vi "MS4_demo.vi"() -> ()   [LabVIEW 2012]
uses:
  <vilib>/vision/Image Controls.llb/IMAQ Image.ctl
  <vilib>/Platform/TimedLoop/XDataNode/timing_clust.ctl
  <vilib>/Platform/TimedLoop/XDataNode/nitl_modes.ctl
  <vilib>/Platform/TimedLoop/XDataNode/wakeup.ctl
  <vilib>/FPGAPlugInAG/sbRIO-9636/niLvFpga_Open_sbRIO-9636.vi
  <vilib>/rvi/interface/common/dynamic/niFpgaDynamicAddResources.vi
  Globals.vi
  <vilib>/Utility/error.llb/Error Cluster From Error Code.vi
  <vilib>/rvi/errors/niLvFpgaAdjustHostInterfaceError.vi
  <vilib>/FPGAPlugInAG/Dynamic/niLvFpga_Close_Dynamic.vi
  <vilib>/platform/TimedLoop/XDataNode/XDataNode.xnode
  <vilib>/rvi/interface/nirviOpenFPGA/nirviOpenFPGA.xnode
  FPGA Bitfiles/NIARC_FPGATarget_FPGACompile_yq6Hl1z977U.lvbitx
  <vilib>/rvi/interface/nirviReadWriteControl/nirviReadWriteControl.xnode
  <vilib>/rvi/interface/nirviCloseFPGA/nirviCloseFPGA.xnode
  <vilib>/Platform/TimedLoop/XDataNode/XDNodeRunTimeDep.lvlib
  NiFpgaLv.dll
  <vilib>/rvi/interface/Simulation/niFpgaSimulationCallBeginRW.vi
panel:
  in  "Go to block?":bool
  out "Arm State":enum16{"arm down", "push", "turn", "arm up"}(ring)
  out "Current \nState":T1(ring)
  in  "Claw deadband":dbl
  in  "Block Claw distance":dbl=0.2
  in  "stop":bool
  in  "Enable":bool
  in  "Block Mid Range":dbl=50.0
  in  "Block Y-Offset":dbl=100.0
  in  "Avoid Distance (m)":dbl=0.3
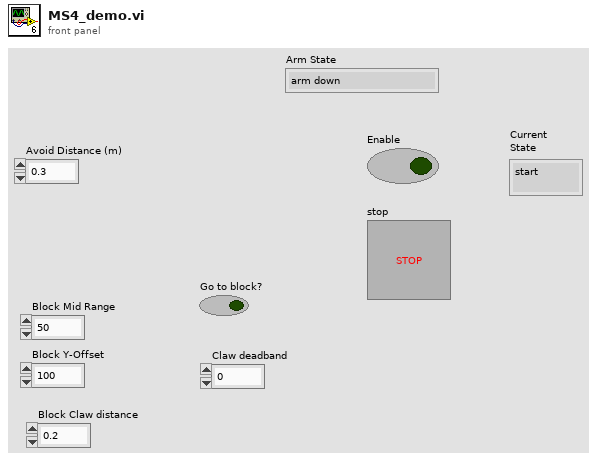
[diagram p1: front panel]
types:
  T1 = enum16{"start", "drive", "turning", "find block", "align block", "pickup"}
  T2 = cluster{"X Velocity (m/s)":dbl, "Y Velocity (m/s)":dbl, "Angular Velocity (rad/s)":dbl}
  T3 = typedef "IMAQ Image.ctl" = refnum<image>
  T4 = typedef "Image Type" = u32
  T5 = enum16{"start", "drive", "turning", "find block", "pickup", ""}
  T6 = enum16{"wait", "open", "close", "lift", "lower", "pickup"}
  T7 = typedef "XDNodeRunTimeDep.lvlib/timing_clust.ctl" = cluster{"Expected End [f-1]":u64, "Actual End [f-1]":u64, "Finished Late? [f-1]":bool, "Expected End [i-1]":u64, "Actual End [i-1]":u64, "Finished Late? [i-1]":bool, "Expected Start [i]":u64, "Actual Start [i]":u64, "Expected Start [f]":u64, "Actual Start [f]":u64, "Source Name":string, "Structure Name":string, "Period":i64, "Deadline":i64, "Offset":i64, "Start":i64, "Priority":i32, "Timeout":i32, "Mode":T8, "Wakeup Reason":T9, "Error":errorcluster, "Source Type":string, "Secondary Source Type":string, "Global End Time":u64, "Global Start Time":u64, "Frame Duration":u64, "Iteration Duration":u64, "Assigned CPU":i32, "I/O Scan Engine Mode":u32}
  T8 = typedef "XDNodeRunTimeDep.lvlib/nitl_modes.ctl" = enum32{"No Change", "Process missed periods, maintain original phase", "Discard missed periods, maintain original phase", "Process missed periods, ignore original phase", "Discard missed periods, ignore original phase"}
  T9 = typedef "XDNodeRunTimeDep.lvlib/wakeup.ctl" = enum32{"Normal", "Aborted", "Asynchronous wakeup", "Timing source error", "Timed loop error", "Timeout"}
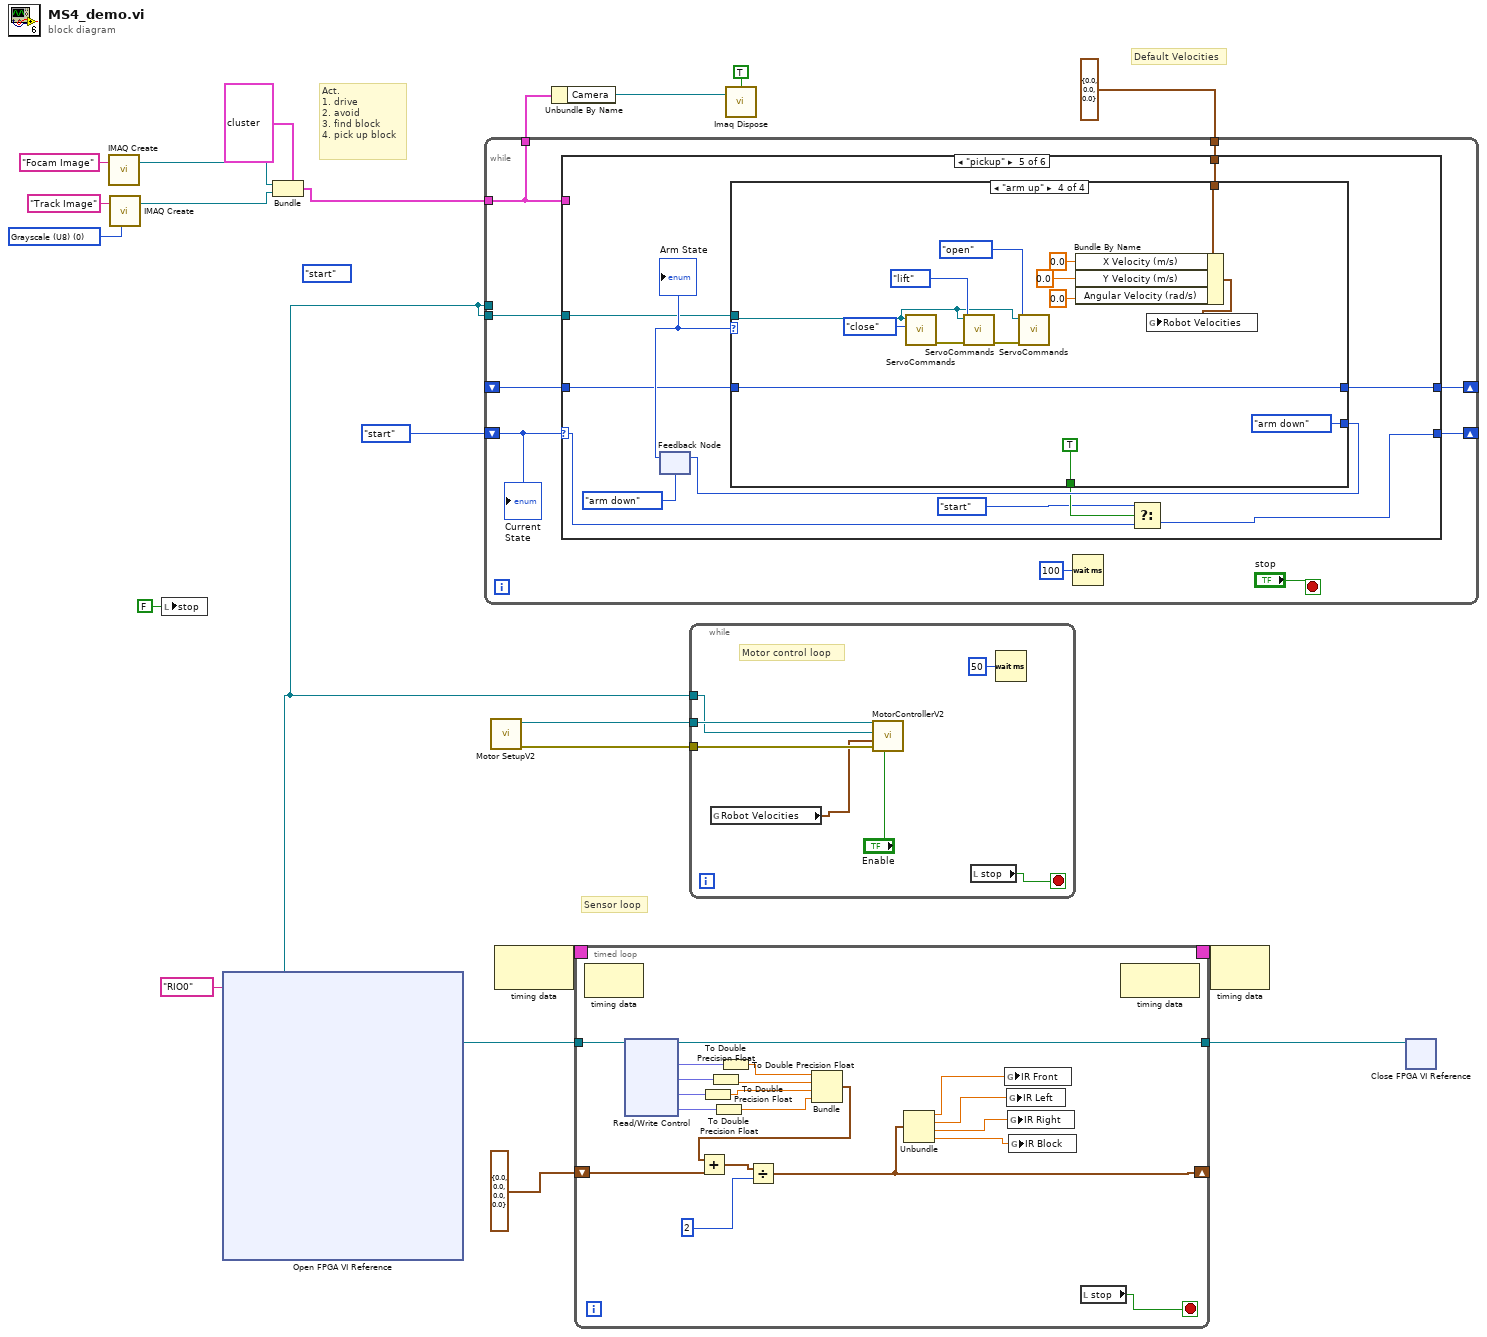
[diagram p0: block diagram]
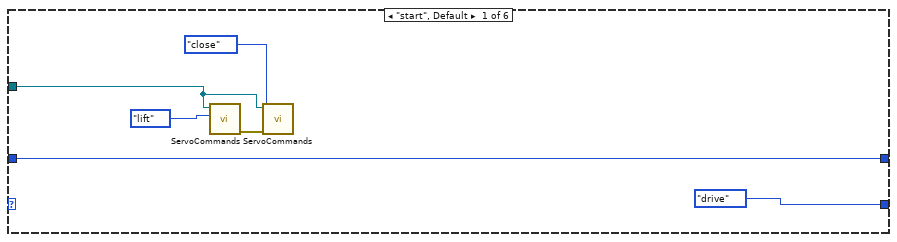
[diagram p2: hidden frame]
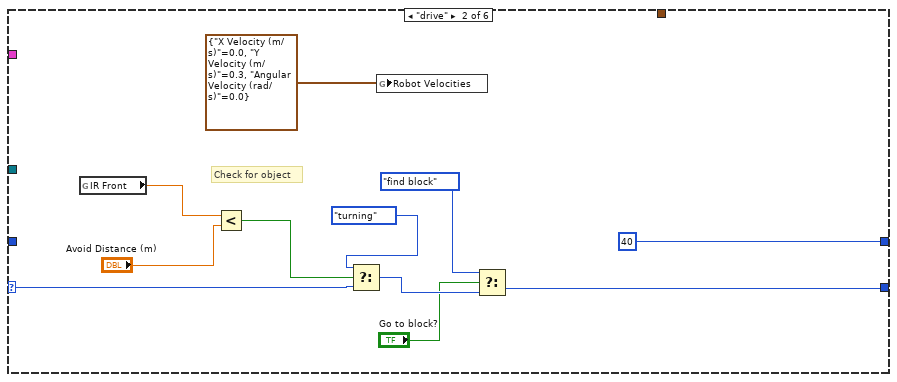
[diagram p3: hidden frame]
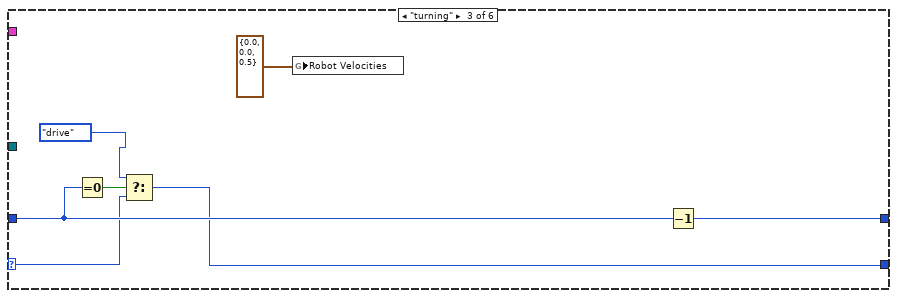
[diagram p4: hidden frame]
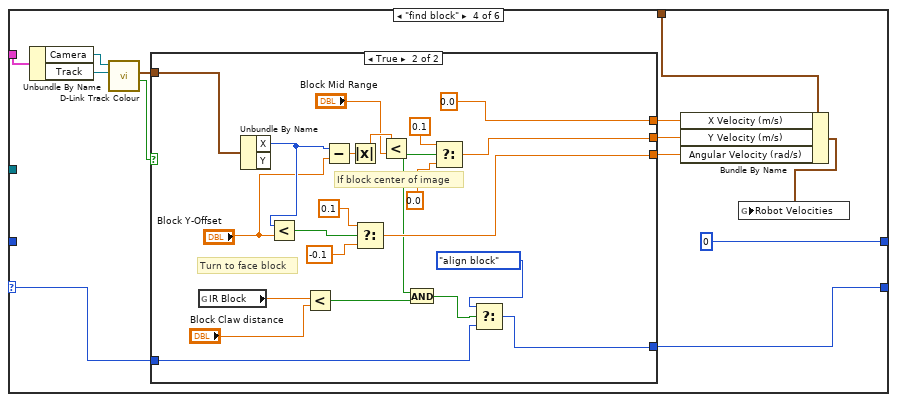
[diagram p5: hidden frame]
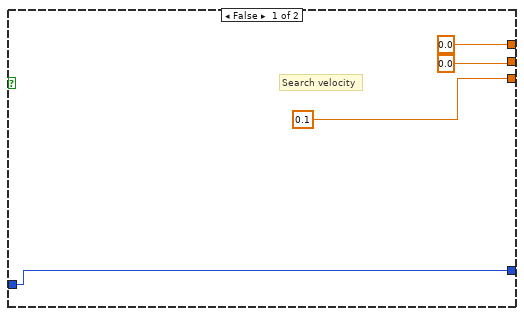
[diagram p6: hidden frame]
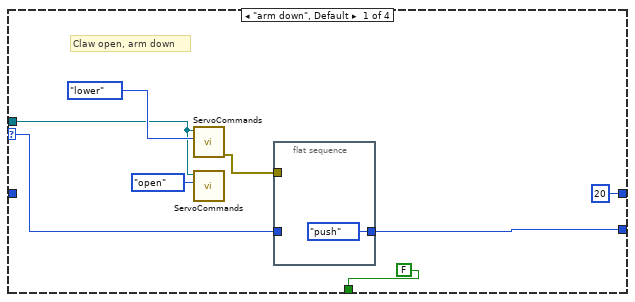
[diagram p7: hidden frame]
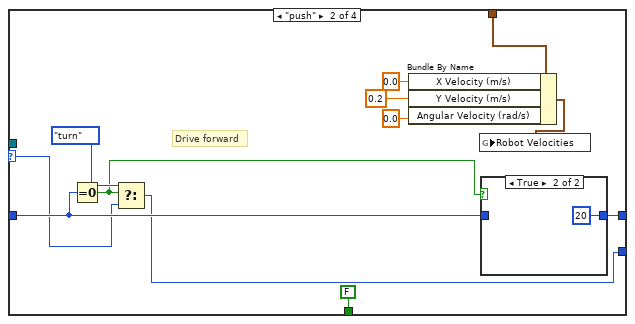
[diagram p8: hidden frame]
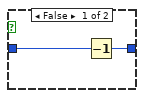
[diagram p9: hidden frame]
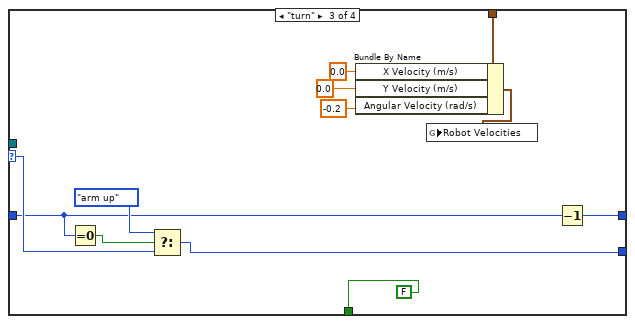
[diagram p10: hidden frame]
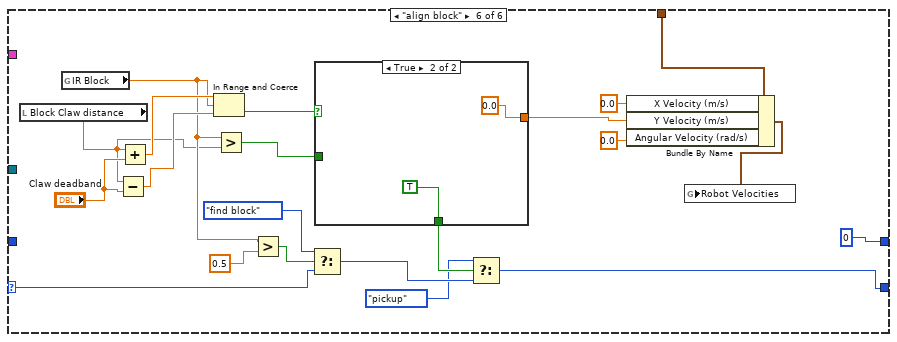
[diagram p11: hidden frame]
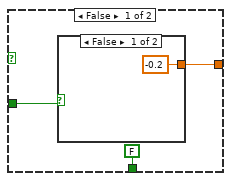
[diagram p12: hidden frame]
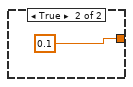
[diagram p13: hidden frame]
diagram:
  w14 = T4 0 items=["Grayscale (U8)", "Grayscale (I16)", "Grayscale (SGL)", "Complex (CSG)", "RGB (U32)", "HSL (U32)", "RGB (U64)", "Grayscale (U16)"] ("Image Type")
  (unwired) T5."start"
  # "Default Velocities"
  # "Sensor loop"
  # "Act.\n1. drive\n2. avoid\n3. find block\n4. pick up block"
  n1 = call "IMAQ Create"("Image Name"="Focam Image") -> ("New Image"=w11:T3)  [unwired: 4 in, 1 out]
  n2 = call "IMAQ Create"("Image Name"="Track Image", "Image Type"=w14) -> ("New Image"=w12:T3)  [unwired: 3 in, 1 out]
  n3 = local write "stop"(FALSE ("stop")) -> ()
  n4 = xnode "Open FPGA VI Reference"("resource name"=tag "RIO0") -> ("FPGA VI Reference Out"=w1:refnum<k20>)  [unwired: 1 in, 1 out]
  n5 = Bundle(cluster=cluster{"Camera":T3, "Track":T3} {"Camera"=refnum, "Track"=refnum}, "Camera"=w11, "Track"=w12) -> (w10:cluster{"Camera":T3, "Track":T3})
  n6 = while {
    tunnel: w1 -> [_]
    shift-right: [w24] -> _
    shift-left: T1."start" -> [w23]
    shift-right: [w30] -> _
    shift-left: _ -> [w29]
    tunnel: w10 -> [w27]
    tunnel: [w27] -> w8
    tunnel: T2 {"X Velocity (m/s)"=0.0, "Y Velocity (m/s)"=0.0, "Angular Velocity (rad/s)"=0.0} ("Robot Velocities") -> [w25]
    tunnel: w1 -> [w22]
    stop <- "stop" stop-if-true
    n7 = case shown="\"pickup\"" w23 {
      selector: w23 -> [_ w44 w51 w56 w97 w161]
      tunnel: [T1."drive" w39 w50 w55 w96 w157] -> w24
      tunnel: [w36 40 w54 0 w100 0] -> w30
      tunnel: w29 -> [w36 _ w53 _ w101 _]
      tunnel: w27 -> [_ _ _ w66 _ _]
      tunnel: w25 -> [_ _ _ w58 w99 w173]
      tunnel: w22 -> [w32 _ _ _ w98 _]
      frame "start", Default {
        n8 = call "ServoCommands.vi"("State"=T6."lift", "FPGA VI Reference In"=w32) -> ("error out"=w33:errorcluster)  [unwired: 9 in]
        n9 = call "ServoCommands.vi"("error in"=w33, "State"=T6."close", "FPGA VI Reference In"=w32) -> ()  [unwired: 8 in, 1 out]
      }
      frame "drive" {
        # "Check for object"
        n10 = global read "Globals.vi" "IR Front"() -> (w47:dbl)
        n11 = Less?(x=w47, y="Avoid Distance (m)") -> (x < y?=w45:bool)
        n12 = Select(t=T1."turning", s=w45, f=w44) -> (s? t:f=w43:T1)
        n13 = global write "Globals.vi" "Robot Velocities"(T2 {"X Velocity (m/s)"=0.0, "Y Velocity (m/s)"=0.3, "Angular Velocity (rad/s)"=0.0} ("Robot Velocities")) -> ()
        n14 = Select(t=T1."find block", s="Go to block?", f=w43) -> (s? t:f=w39:T1)
      }
      frame "turning" {
        n15 = Equal To 0?(x=w53) -> (x = 0?=w52:bool)
        n16 = Select(t=T1."drive", s=w52, f=w51) -> (s? t:f=w50:T1)
        n17 = global write "Globals.vi" "Robot Velocities"(T2 {"X Velocity (m/s)"=0.0, "Y Velocity (m/s)"=0.0, "Angular Velocity (rad/s)"=0.5} ("Robot Velocities")) -> ()
        n18 = Decrement(x=w53) -> (x-1=w54:i32)
      }
      frame "find block" {
        n19 = Unbundle By Name(w66) -> ("Camera"=w65:T3, "Track"=w64:T3)
        n20 = call "D-Link Track Colour.vi"("Image Dst"=w64, "New Image"=w65) -> ("Object found?"=w57:bool, "Object Output"=w59:cluster{"X":i32, "Y":i32})  [unwired: 7 in, 1 out]
        n21 = case shown="True" w57 {
          tunnel: [0.0 ("X Velocity (m/s)") 0.0 ("X Velocity (m/s)")] -> w63
          tunnel: [0.1 ("f") w92] -> w62
          tunnel: [0.0 ("f") w88] -> w61
          tunnel: w59 -> [_ w82]
          tunnel: [w68 w75] -> w55
          tunnel: w56 -> [w68 w76]
          frame False {
            # "Search velocity"
          }
          frame True {
            # "Turn to face block"
            # "If block center of image"
            n22 = global read "Globals.vi" "IR Block"() -> (w81:dbl)
            n23 = Unbundle By Name(w82) -> ("X"=w85:i32)  [unwired: 1 out]
            n24 = Less?(x=w85, y="Block Y-Offset") -> (x < y?=w89:bool)
            n25 = Less?(x=w81, y="Block Claw distance") -> (x < y?=w78:bool)
            n26 = Subtract(x=w85, y="Block Y-Offset") -> (x-y=w83:dbl)
            n27 = Absolute Value(x=w83) -> (abs(x)=w74:dbl)
            n28 = Select(t=0.1, s=w89, f=-0.1) -> (s? t:f=w92:dbl)
            n29 = Less?(x=w74, y="Block Mid Range") -> (x < y?=w79:bool)
            n30 = And(x=w79, y=w78) -> (x .and. y?=w77:bool)
            n31 = Select(t=0.1, s=w79, f=0.0) -> (s? t:f=w88:dbl)
            n32 = Select(t=T1."align block", s=w77, f=w76) -> (s? t:f=w75:T1)
          }
        }
        n33 = Bundle By Name(cluster=w58, "X Velocity (m/s)"=w63, "Y Velocity (m/s)"=w61, "Angular Velocity (rad/s)"=w62) -> (w60:T2)
        n34 = global write "Globals.vi" "Robot Velocities"(w60) -> ()
      }
      frame "pickup" {
        n35 = feedback #1(enum16{"arm down", "push", "turn", "arm up"}."arm down") -> (w102:enum16{"arm down", "push", "turn", "arm up"})
        "Arm State" <- w102
        n36 = case shown="\"arm up\"" w102 {
          selector: w102 -> [w107 w119 w140 _]
          tunnel: [w108 w118 w133 enum16{"arm down", "push", "turn", "arm up"}."arm down" ("t")] -> w104
          tunnel: w101 -> [_ w120 w131 w154]
          tunnel: [20 w121 w139 w154] -> w100
          tunnel: w99 -> [_ w122 w135 w149]
          tunnel: w98 -> [w110 _ _ w141]
          tunnel: [FALSE FALSE FALSE TRUE] -> w95
          frame "arm down", Default {
            # "Claw open, arm down"
            n37 = call "ServoCommands.vi"("State"=T6."lower", "FPGA VI Reference In"=w110) -> ("error out"=w106:errorcluster)  [unwired: 9 in]
            n38 = call "ServoCommands.vi"("State"=T6."open", "FPGA VI Reference In"=w110) -> ()  [unwired: 9 in, 1 out]
            n39 = flat-sequence {
              tunnel: [enum16{"arm down", "push", "turn", "arm up"}."push"] -> w108
              tunnel: w107 -> [_]
              tunnel: w106 -> [_]
              frame #0 {
              }
            }
          }
          frame "push" {
            # "Drive forward"
            n40 = Equal To 0?(x=w120) -> (x = 0?=w116:bool)
            n41 = Select(t=enum16{"arm down", "push", "turn", "arm up"}."turn", s=w116, f=w119) -> (s? t:f=w118:enum16{"arm down", "push", "turn", "arm up"})
            n42 = Bundle By Name(cluster=w122, "X Velocity (m/s)"=0.0, "Y Velocity (m/s)"=0.2, "Angular Velocity (rad/s)"=0.0) -> (w125:T2)
            n43 = global write "Globals.vi" "Robot Velocities"(w125) -> ()
            n44 = case shown="True" w116 {
              tunnel: [w127 20] -> w121
              tunnel: w120 -> [w126 _]
              frame False {
                n45 = Decrement(x=w126) -> (x-1=w127:i32)
              }
              frame True {
              }
            }
          }
          frame "turn" {
            n46 = Equal To 0?(x=w131) -> (x = 0?=w130:bool)
            n47 = Select(t=enum16{"arm down", "push", "turn", "arm up"}."arm up", s=w130, f=w140) -> (s? t:f=w133:enum16{"arm down", "push", "turn", "arm up"})
            n48 = Bundle By Name(cluster=w135, "X Velocity (m/s)"=0.0, "Y Velocity (m/s)"=0.0, "Angular Velocity (rad/s)"=-0.2) -> (w138:T2)
            n49 = global write "Globals.vi" "Robot Velocities"(w138) -> ()
            n50 = Decrement(x=w131) -> (x-1=w139:i32)
          }
          frame "arm up" {
            n51 = call "ServoCommands.vi"("State"=T6."close", "FPGA VI Reference In"=w141) -> ("error out"=w147:errorcluster)  [unwired: 9 in]
            n52 = call "ServoCommands.vi"("error in"=w147, "State"=T6."lift", "FPGA VI Reference In"=w141) -> ("error out"=w143:errorcluster)  [unwired: 8 in]
            n53 = call "ServoCommands.vi"("error in"=w143, "State"=T6."open", "FPGA VI Reference In"=w141) -> ()  [unwired: 8 in, 1 out]
            n54 = Bundle By Name(cluster=w149, "X Velocity (m/s)"=0.0, "Y Velocity (m/s)"=0.0, "Angular Velocity (rad/s)"=0.0) -> (w153:T2)
            n55 = global write "Globals.vi" "Robot Velocities"(w153) -> ()
          }
        }
        n56 = feedback-in #1(w104) -> ()
        n57 = Select(t=T1."start", s=w95, f=w97) -> (s? t:f=w96:T1)
      }
      frame "align block" {
        n58 = local read "Block Claw distance"() -> (w155:dbl)
        n59 = global read "Globals.vi" "IR Block"() -> (w164:dbl)
        n60 = Subtract(x=w155, y="Claw deadband") -> (x-y=w166:dbl)
        n61 = Add(x=w155, y="Claw deadband") -> (x+y=w169:dbl)
        n62 = In Range and Coerce(upper limit=w169, x=w164, lower limit=w166) -> (In Range?=w168:bool)  [unwired: 1 out]
        n63 = Greater?(x=w164, y=w155) -> (0:w165:bool)
        n64 = Greater?(x=w164, y=0.5) -> (0:w162:bool)
        n65 = Select(t=T1."find block", s=w162, f=w161) -> (s? t:f=w158:T1)
        n66 = case shown="True" w168 {
          tunnel: [w178 0.0 ("Y Velocity (m/s)")] -> w170
          tunnel: w165 -> [w177 _]
          tunnel: [FALSE TRUE] -> w159
          frame False {
            n67 = case shown="False" w177 {
              tunnel: [-0.2 ("Y Velocity (m/s)") 0.1 ("Y Velocity (m/s)")] -> w178
              frame False {
              }
              frame True {
              }
            }
          }
          frame True {
          }
        }
        n68 = Select(t=T1."pickup", s=w159, f=w158) -> (s? t:f=w157:T1)
        n69 = Bundle By Name(cluster=w173, "X Velocity (m/s)"=0.0, "Y Velocity (m/s)"=w170, "Angular Velocity (rad/s)"=0.0) -> (w174:T2)
        n70 = global write "Globals.vi" "Robot Velocities"(w174) -> ()
      }
    }
    n71 = Wait (ms)(milliseconds to wait=u32 100) -> ()  [unwired: 1 out]
    "Current \nState" <- w23
  }
  n72 = call "Motor SetupV2.vi"() -> ("error out"=w20:errorcluster, "mecanum steering frame out"=w21:refnum<class "NI_Robotics_Mecanum Steering Frame.lvclass">)  [unwired: 10 in]
  n73 = node-c288() -> (w19:T7)  [unwired: 1 in]
  n74 = Unbundle By Name(w8) -> ("Camera"=w7:T3)
  n75 = timed-loop {
    timing: w19 -> [_]
    timing-out: [_] -> w18
    tunnel: w1 -> [w202]
    shift-right: [w191] -> _
    shift-left: cluster{dbl, dbl, dbl, dbl} {0.0, 0.0, 0.0, 0.0} -> [w195]
    tunnel: [w186] -> w4
    stop <- w187 stop-if-true
    n76 = node-c288() -> ()  [unwired: 1 in, 1 out]
    n77 = xnode "Read/Write Control"("FPGA VI Reference In"=w202) -> ("FPGA VI Reference Out"=w186:refnum<k20>, "IR 0"=w201:fxp<+/-,24,5>, "IR 1"=w200:fxp<+/-,24,5>, "IR 2"=w199:fxp<+/-,24,5>, "IR 3"=w185:fxp<+/-,24,5>)  [unwired: 1 in, 1 out]
    n78 = To Double Precision Float(number=w199) -> (double precision float=w196:dbl)
    n79 = To Double Precision Float(number=w200) -> (double precision float=w197:dbl)
    n80 = To Double Precision Float(number=w185) -> (double precision float=w184:dbl)
    n81 = To Double Precision Float(number=w201) -> (double precision float=w198:dbl)
    n82 = Bundle(w198, w197, w196, w184) -> (w194:cluster{dbl, dbl, dbl, dbl})  [unwired: 1 in]
    n83 = Add(x=w194, y=w195) -> (x+y=w193:cluster{dbl, dbl, dbl, dbl})
    n84 = Divide(x=w193, y=2) -> (x/y=w191:cluster{dbl, dbl, dbl, dbl})
    n85 = Unbundle(w191) -> (w190:dbl, w189:dbl, w188:dbl, w183:dbl)
    n86 = global write "Globals.vi" "IR Front"(w190) -> ()
    n87 = global write "Globals.vi" "IR Left"(w189) -> ()
    n88 = global write "Globals.vi" "IR Right"(w188) -> ()
    n89 = global write "Globals.vi" "IR Block"(w183) -> ()
    n90 = local read "stop"() -> (w187:bool)
    n91 = node-c288() -> ()  [unwired: 1 in, 1 out]
  }
  n92 = while {
    tunnel: w21 -> [w211]
    tunnel: w20 -> [w210]
    tunnel: w1 -> [w209]
    stop <- w205 stop-if-true
    # "Motor control loop"
    n93 = global read "Globals.vi" "Robot Velocities"() -> (w208:T2)
    n94 = call "MotorControllerV2.vi"("Enable"="Enable", "error in"=w210, "Robot Velocities"=w208, "FPGA VI Reference In"=w209, "mecanum steering frame in"=w211) -> ()  [unwired: 5 in, 2 out]
    n95 = local read "stop"() -> (w205:bool)
    n96 = Wait (ms)(milliseconds to wait=u32 50) -> ()  [unwired: 1 out]
  }
  n97 = call "Imaq Dispose"("All Images? (No)"=TRUE, "Image"=w7) -> ()  [unwired: 4 in, 1 out]
  n98 = node-c288(w18) -> ()  [unwired: 1 out]
  n99 = xnode "Close FPGA VI Reference"("FPGA VI Reference In"=w4) -> ()  [unwired: 1 in, 1 out]
